vi "ANDOR_GetDetector.vi"(8 "error in (no error)":errorcluster) -> (0 "error out":errorcluster, 1 "DLL error code":u32, 2 "ypixels":i32, 3 "xpixels":i32, 5 "Detector Size":i32[](array[numeric]))   [LabVIEW 2010]
doc: "This function returns the size of the detector in pixels. The horizontal axis is taken to be the axis parallel to the readout register.\n\n<B>Parameters:</B>\nxpixels - number of horizontal pixels\nypixels - number of vertical pixels\n\n<B>Error codes:</B>\nDRV_SUCCESS - Detector size returned.\nDRV_NOT_INITIALIZED - System not initialized.\nDRV_ACQUIRING - Acquisition in progress."
uses:
  Program Files/Andor SOLIS/atmcd32d.dll
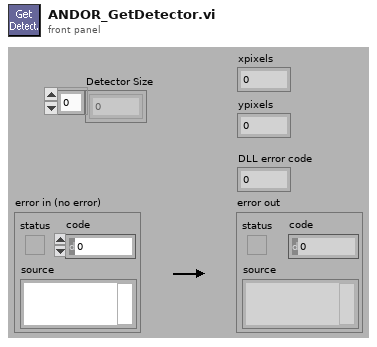
[diagram p1: front panel]
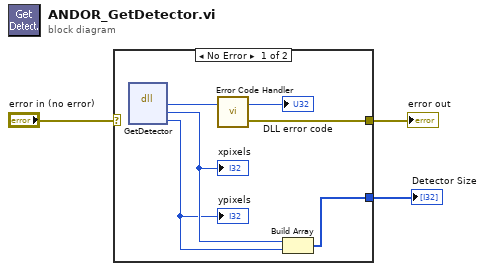
[diagram p0: block diagram]
diagram:
  n1 = case shown="No Error" "error in (no error)" {
    selector: "error in (no error)" -> [_ w10]
    tunnel: [w8 w10] -> w2
    tunnel: [w4 _] -> w1
    frame No Error {
      n2 = dll-call lib="C:/Program Files/Andor SOLIS/atmcd32d.dll" fn="GetDetector"() -> ("return type"=w9:u32, "xpixels"=w6:i32, "ypixels"=w5:i32)  [unwired: 3 in, 4 out]
      "xpixels" <- w6
      "ypixels" <- w5
      n3 = call <userlib>:"Error Code Handler.vi"("DLL error code"=w9) -> ("error out"=w8:errorcluster, "dup DLL error code"=→"DLL error code":u32)  [unwired: 1 out]
      n4 = Build Array(w6, w5) -> (w4:i32[])
    }
    frame Error {
    }
  }
  "error out" <- w2
  "Detector Size" <- w1
